vi "PCAN_READ.vi"(8 "error in (no error)":errorcluster) -> (0 "error out":errorcluster, 2 "TPCANMsg":T2 {"ID" format="%x"; "MSGTYPE" items=["STATUS"=128, "EXTENDED"=2, "RTR"=1, "DATA MSG"=0]; "aDATA" format="%x"}, 3 "error":T1 items=["CAN_ERR_OK"=0, "CAN_ERR_XMTFULL"=1, "CAN_ERR_OVERRUN"=2, "CAN_ERR_BUSLIGHT"=4, "CAN_ERR_BUSHEAVY"=8, "CAN_ERR_BUSOFF"=16, "CAN_ERR_QRCVEMPTY"=32, "CAN_ERR_QOVERRUN"=64, "CAN_ERR_QXMTFULL"=128, "CAN_ERR_REGTEST"=256, "CAN_ERR_NOVXD"=512, "CAN_ERR_RESOURCE"=8192, "CAN_ERR_ILLPARAMTYPE"=16384, "CAN_ERR_ILLPARAMVAL"=32768])   [LabVIEW 2016]
doc: "///////////////////////////////////////////////////////////////////////////////\n// CAN_Read()\n// gibt die naechste Message oder den naechsten Fehler aus dem\n// RCV-Queue des Clients zurueck.\n//\n// CAN_Read() gibt die nächste Message oder den nächsten Fehler aus dem RCV-Queue des Clients zurück. Message wird\n// nach 'msgbuff' geschrieben. ACHTUNG der MSG_Type gibt an ob es sich um eine 11Bit, 29Bit, RTR oder Status\n// Nachricht handelt. IMMER abfragen !. \n// \n// Ist die gelesene CAN Nachricht keine normale Nachricht sondern eine Statusmeldung so ist der Rueckgabewert \n// der CAN_Read() Funktion weiterhin CAN_ERR_OK, jedoch ist in TPCAN_MSG Struktur der MSGTYPE = MSGTYPE_STATUS.\n// \n// Identifier und Laegencode einer solchen Statusnachricht duerfen nicht ausgewertet werden (undefinierte Werte).\n// Die eigentliche Information ueber den Fehler lassen sich nun aus den ersten 4 Datenbytes der Nachricht \n// herauslesen:\n// \n// Data0 Data1 Data2 Data3 Fehlertyp\n// 0x00 0x00 0x00 0x02 == CAN_ERR_OVERRUN 0x0002 // CAN-Controller wurde zu spaet gelesen\n// 0x00 0x00 0x00 0x04 == CAN_ERR_BUSLIGHT 0x0004 // Busfehler: ein Errorcounter erreichte Limit (96)\n// 0x00 0x00 0x00 0x08 == CAN_ERR_BUSHEAVY 0x0008 // Busfehler: ein Errorcounter erreichte Limit (128)\n// \n// 0x00 0x00 0x00 0x10 == CAN_ERR_BUSOFF 0x0010 // Busfehler: CAN_Controller ging 'Bus-Off'\n// \n// Beim Empfangen einer BUSOFF Statusnachricht ist der CAN-Controller mit CAN_Init() neu zu initialisieren,\n// da sonst keine Nachrichtem mehr gesendet werden koennen!\n// \n// \n// Message wird nach 'msgbuff' geschrieben.\n// moegliche Fehler: NOVXD QRCVEMPTY\n//\n\nDWORD __stdcall CAN_Read(TPCANMsg* pMsgBuff );"
uses:
  PCAN_ERROR.ctl
  PCAN_USB.DLL
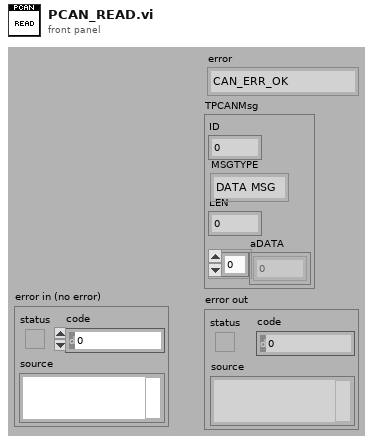
[diagram p1: front panel]
types:
  T1 = typedef "PCAN_ERROR.ctl" = i32
  T2 = cluster{"ID":u32, "MSGTYPE":u8, "LEN":u8, "aDATA":u8[]}
  T3 = enum16{"big-endian, network order", "native, host order", "little-endian"}
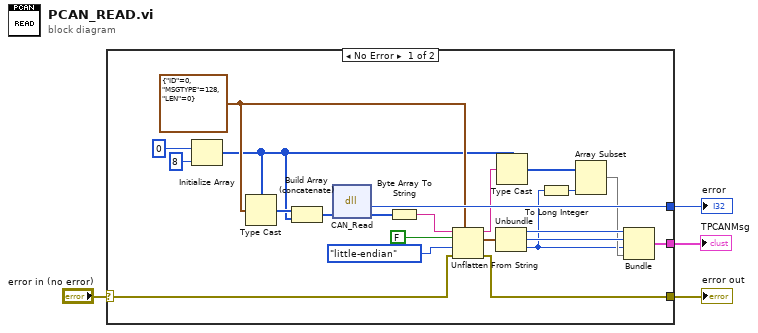
[diagram p0: block diagram]
diagram:
  n1 = case shown="No Error" "error in (no error)" {
    selector: "error in (no error)" -> [w17 w27]
    tunnel: [w26 _] -> w1
    tunnel: [w24 w27] -> w3
    tunnel: [w12 _] -> w2
    frame No Error {
      w18 = cluster{"ID":u32, "MSGTYPE":u8, "LEN":u8} {"ID"=0, "MSGTYPE"=128, "LEN"=0} ("TPCANMsg")
      n2 = Initialize Array(u8 0 ("DATA"), 8 ("dimension size")) -> (w14:u8[])
      n3 = Type Cast(type=w14, x=w18) -> (*(type *) &x=w15:u8[])
      n4 = Build Array (concatenate)(w15, w14) -> (w13:u8[])
      n5 = dll-call lib="D:/LabView/08_PCAN&Measurement/PCAN_Driver/PCAN_USB.DLL" fn="CAN_Read"("pMsgBuff"=w13) -> ("return type"=w26:i32, "pMsgBuff"=w23:u8[])  [unwired: 3 in, 2 out]
      n6 = Byte Array To String(unsigned byte array=w23) -> (string=w25:string)
      n7 = Unflatten From String(type=w18, binary string=w25, data includes array or string size? (T)=FALSE ("prepend array or string size? (T)"), byte order (0:big-endian, network order)=T3."little-endian", error in (no error)=w17) -> (rest of the binary string=w16:string, value=w11:cluster{"ID":u32, "MSGTYPE":u8, "LEN":u8}, error out=w24:errorcluster)
      n8 = Unbundle(w11) -> ("ID"=w9:u32, "MSGTYPE"=w10:u8, "LEN"=w5:u8)
      n9 = Type Cast(type=w14, x=w16) -> (*(type *) &x=w7:u8[])
      n10 = To Long Integer(number=w5) -> (32bit integer=w8:i32)
      n11 = Array Subset(array=w7, length=w8) -> (w6:u8[])  [unwired: 1 in]
      n12 = Bundle("ID"=w9, "MSGTYPE"=w10, "LEN"=w5, w6) -> (w12:cluster{"ID":u32, "MSGTYPE":u8, "LEN":u8, u8[]})  [unwired: 1 out]
    }
    frame Error {
    }
  }
  "error out" <- w3
  "TPCANMsg" <- w2
  "error" <- w1
